vi "Input Control.vi"(2 "Controller":T1, 3 "State":enum16{"Open", "Run", "End"}(ring)) -> (0 "Buttons":T2, 1 "Axes":T3)   [LabVIEW 2013]
uses:
  <vilib>/Rock Robotics/WPI/Joystick/WPI_JoystickButtonState.ctl
  <vilib>/Rock Robotics/WPI/Joystick/WPI_JoystickDeviceEnum.ctl
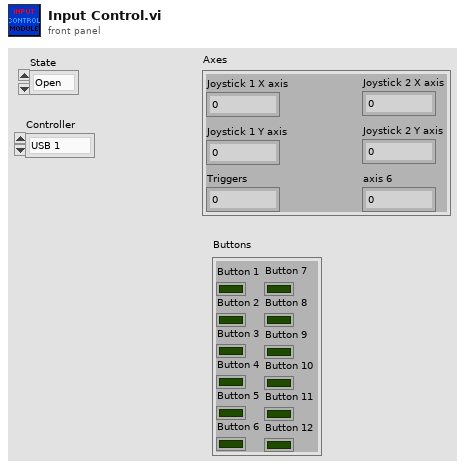
[diagram p1: front panel]
types:
  T1 = typedef "WPI_JoystickDeviceEnum.ctl" = enum16{"USB 1", "USB 2", "USB 3", "USB 4", "Kinect 1", "Kinect 2"}
  T2 = typedef "WPI_JoystickButtonState.ctl" = cluster{"Button 1":bool, "Button 2":bool, "Button 3":bool, "Button 4":bool, "Button 5":bool, "Button 6":bool, "Button 7":bool, "Button 8":bool, "Button 9":bool, "Button 10":bool, "Button 11":bool, "Button 12":bool}
  T3 = cluster{"Joystick 1 X axis":dbl, "Joystick 1 Y axis":dbl, "Triggers":dbl, "Joystick 2 X axis":dbl, "Joystick 2 Y axis":dbl, "axis 6":dbl}
  T4 = typedef "WPI_JoystickDevRef.ctl" = cluster{"Device":T1}
  T5 = cluster{"axis 1 (x)":dbl, "axis 2 (y)":dbl, "axis 3 (throttle)":dbl, "axis 4":dbl, "axis 5":dbl, "axis 6":dbl}
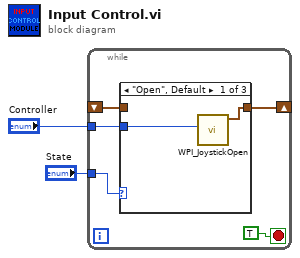
[diagram p0: block diagram]
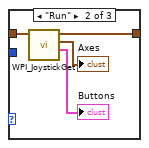
[diagram p2: hidden frame]
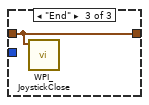
[diagram p3: hidden frame]
diagram:
  n1 = while {
    tunnel: "State" -> [w7]
    shift-right: [w6] -> _
    shift-left: _ -> [w5]
    tunnel: "Controller" -> [w3]
    stop <- TRUE stop-if-true
    n2 = case shown="\"Open\", Default" w7 {
      tunnel: [w9 w12 w14] -> w6
      tunnel: w5 -> [_ w13 w14]
      tunnel: w3 -> [w8 _ _]
      frame "Open", Default {
        n3 = call <vilib>:"WPI_JoystickOpen.vi"("JoystickDevice"=w8) -> ("JoystickDevRef"=w9:T4)  [unwired: 10 in]
      }
      frame "Run" {
        n4 = call <vilib>:"WPI_JoystickGet.vi"("JoystickDevRef"=w13) -> ("Buttons"=→"Buttons":T2, "Axes"=→"Axes":T5, "JoystickDevRef"=w12:T4)  [unwired: 4 in]
      }
      frame "End" {
        n5 = call <vilib>:"WPI_JoystickClose.vi"("JoystickDevRef"=w14) -> ()  [unwired: 11 in]
      }
    }
  }
